vi "Close Web Service.vi"(8 "error in (no error)":errorcluster, 11 "CheckPqmNtrsAndProductSerialDateService refnum":refnum<k24>) -> (0 "error out":errorcluster)   [LabVIEW 2023, in "CheckPqmNtrsAndProductSerialDateService.lvlib"]
uses:
  <userlib>/WebService/_CheckPqmNtrsAndProductSerialDateService/CheckPqmNtrsAndProductSerialDateService.dll
  <userlib>/WebService/_CheckPqmNtrsAndProductSerialDateService/CheckPqmNtrsAndProductSerialDateService.lvlib
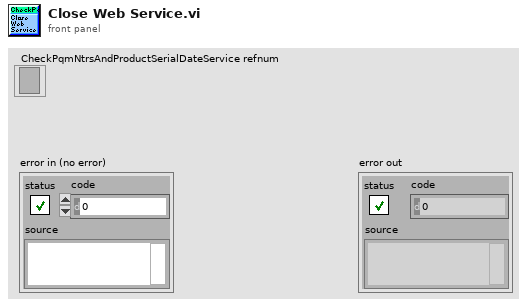
[diagram p1: front panel]
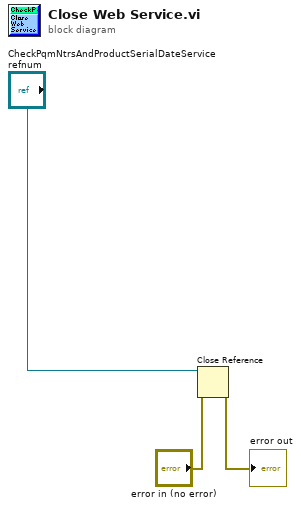
[diagram p0: block diagram]
diagram:
  n1 = Close Reference(reference="CheckPqmNtrsAndProductSerialDateService refnum", error in (no error)="error in (no error)") -> (error out=→"error out":errorcluster)
